vi "CheckOneTouchShot.vi"(0 "Utilities in":refnum<class "Utilities.lvclass">, 5 "Point":dbl[](array[numeric]), 7 "Best y":dbl, 9 "GameRef":refnum<data-value>, 11 "error in (no error)":errorcluster, 12 "Ally?":bool) -> (4 "Utilities out":refnum<class "Utilities.lvclass">, 6 "OneTouch":bool, 10 "Angle":dbl, 15 "error out":errorcluster)   [LabVIEW 2023, in "Utilities.lvclass"]
uses:
  Utilities.lvclass
  Game_class/Game.lvclass
  Game_class/Game.lvclass/Game.ctl
  Field_class/Field.lvclass/Field.ctl
  Object_class/Object.lvclass/Object.ctl
  Game_class/Read FieldRef.vi
  Game_class/Read BallRef.vi
  Object_class/Read position(x,y).vi
  Field_class/Read enemyGoalPosition.vi
  Field_class/Read ourGoalPosition.vi
  Ball_class/Ball.lvclass
  C:/Users/ebert/Documents/codes/SSL/repo/SSL_AI/Object_class/Object.lvclass
  Field_class/Field.lvclass
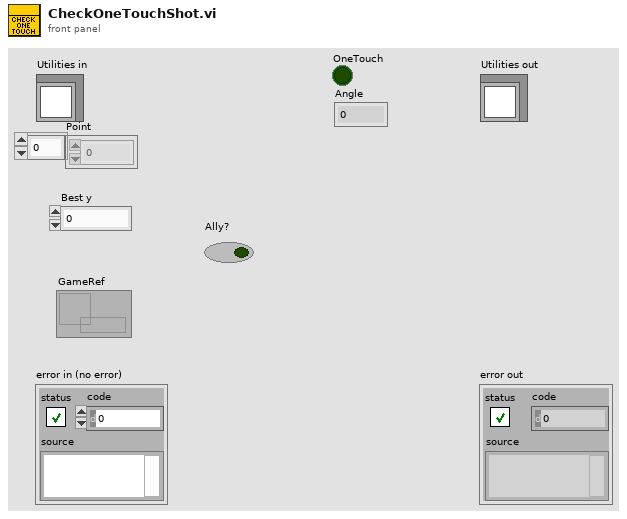
[diagram p1: front panel]
types:
  T1 = typedef "STPParameters.ctl" = cluster{"Skills":T2, "TestSkill":T4, "Events":cluster{"distanceToBallPossession":dbl, "timeForPossessionThreshold":dbl}, "Criteria":cluster{"OpenAngleToGoal":cluster{"minAngle":dbl, "maxAngle":dbl, "minEvaluation":dbl}, "PassDistance":cluster{"maxDistance":dbl, "minDistance":dbl}, "ShotInterception":cluster{"shotSpeed":dbl, "minEnemySpeed":dbl, "minEvaluation":dbl, "maxEnemySpeed":dbl}, "OneTouchShot":cluster{"MaxAngle":dbl, "minEvaluation":dbl}, "PassInterception":cluster{"minEnemySpeed":dbl, "maxEnemySpeed":dbl, "chipPassDistance":dbl, "chipPassEval":dbl, "minEvaluation":dbl}}, "minPassSpeed":dbl, "maxPassSpeed":dbl, "AllyTeamIds":T5[], "ReceiverSpeed":dbl, "minEvaluationToShoot":dbl, "maxDefendersNumber":u8}
  T2 = typedef "Skills.ctl" = cluster{"CirculateBall":T3, "ProtectBall":cluster{"DistanceFromBall":dbl}}
  T3 = typedef "CIrculateSkillParameters.ctl" = cluster{"rotationAngle":dbl, "velocityFactor":dbl, "OrientationFactor":dbl}
  T4 = typedef "TestSkills.ctl" = enum16{"AlignSkill", "PassSkill", "CirculateBall", "OneTouchShotSkill", "KickToSkill_v2", "ShootSkill", "InterceptBall", "Exit", "GoToSkill_v2"}
  T5 = typedef "AllyTeam.ctl" = enum16{"Keeper", "Defender", "Attacker"}
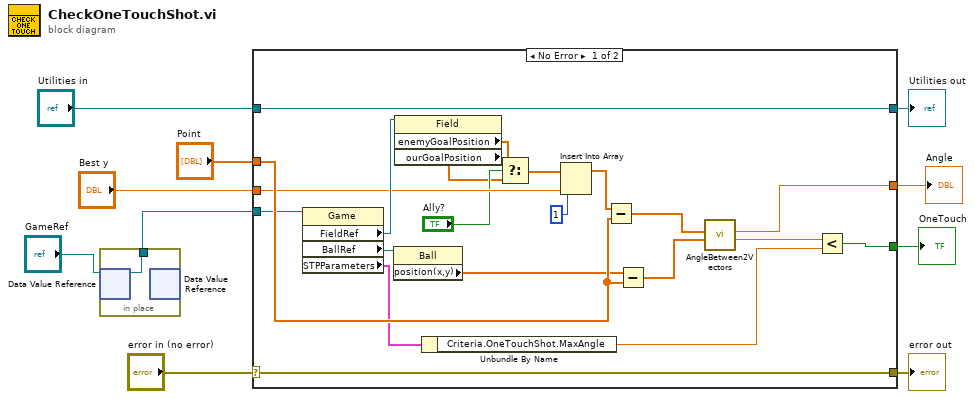
[diagram p0: block diagram]
diagram:
  n1 = in-place {
    in-place-border: [w11] -> w2
    n2 = in-place-dvr #1("GameRef") -> (w11:refnum<class "Game.lvclass">)  [unwired: 1 out]
    n3 = in-place-dvr #1() -> ()  [unwired: 1 in, 2 out]
  }
  n4 = case shown="No Error" "error in (no error)" {
    selector: "error in (no error)" -> [w32 w34]
    tunnel: [w32 w34] -> w9
    tunnel: [w31 w33] -> w7
    tunnel: "Utilities in" -> [w31 w33]
    tunnel: "Point" -> [w26 _]
    tunnel: [w23 _] -> w5
    tunnel: "Best y" -> [w22 _]
    tunnel: w2 -> [w17 _]
    tunnel: [w12 _] -> w1
    frame No Error {
      n5 = property class="Game"(reference=w17) -> ("FieldRef"=w30:refnum<class "Field.lvclass">, "BallRef"=w27:refnum<class "Ball.lvclass">, "STPParameters"=w24:T1)  [unwired: 1 in, 2 out]
      n6 = property class="Ball"(reference=w27) -> ("position(x,y)"=w25:dbl[])  [unwired: 1 in, 2 out]
      n7 = property class="Field"(reference=w30) -> ("enemyGoalPosition"=w19:dbl[], "ourGoalPosition"=w18:dbl[])  [unwired: 1 in, 2 out]
      n8 = Unbundle By Name(w24) -> ("Criteria.OneTouchShot.MaxAngle"=w14:dbl)
      n9 = Select(t=w19, s="Ally?", f=w18) -> (s? t:f=w21:dbl[])
      n10 = Insert Into Array(array=w21, index=1, new element=w22) -> (w28:dbl[])
      n11 = Subtract(x=w28, y=w26) -> (x-y=w16:dbl[])
      n12 = Subtract(x=w25, y=w26) -> (x-y=w15:dbl[])
      n13 = call "AngleBetween2Vectors.vi"("Array 1"=w15, "Array 2"=w16) -> ("angleInDegrees"=w13:dbl, "angleInRadians(default)"=w12:dbl)  [unwired: 6 in, 2 out]
      n14 = Less?(x=w13, y=w14) -> (x < y?=w23:bool)
    }
    frame Error {
    }
  }
  "error out" <- w9
  "Utilities out" <- w7
  "OneTouch" <- w5
  "Angle" <- w1
